vi "Listener.vi"(8 "error in (no error)":errorcluster, 11 "Hitronics in":refnum<class "Hitronics.lvclass">) -> (0 "error out":errorcluster, 2 "Buffer Dump":string, 3 "Hitronics out":refnum<class "Hitronics.lvclass">)   [LabVIEW 2018, in "Hitronics.lvlib" / "Hitronics.lvclass"]
uses:
  Hitronics.lvclass
  PPLs/Laser/Parent/Laser.lvlibp/Laser.lvclass
  C:/AME Test Engineering/LabVIEW/PPLs/Laser/Parent/Laser.lvlibp/Laser.lvclass
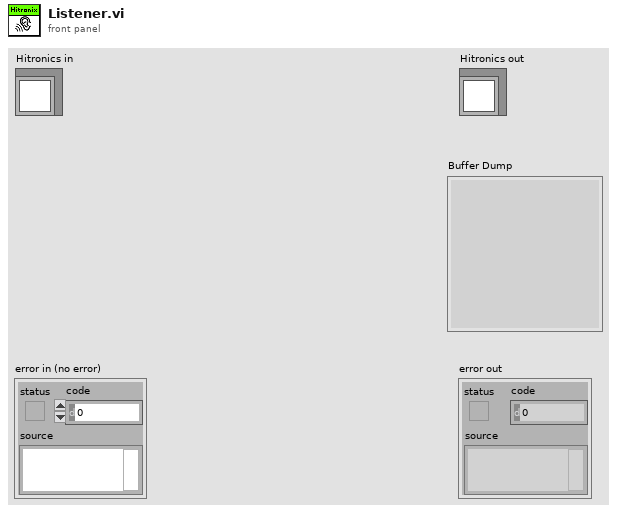
[diagram p1: front panel]
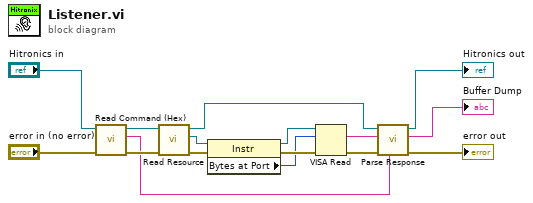
[diagram p0: block diagram]
diagram:
  n1 = call-dynamic "Read Command (Hex).vi"("error in (no error)"="error in (no error)", "Hitronics in"="Hitronics in") -> ("error out"=w13:errorcluster, "Command (Hex)"=w5:string, "Hitronics out"=w14:refnum<class "Hitronics.lvclass">)  [unwired: 7 in]
  n2 = call "Read Resource.vi"("error in (no error)"=w13, "Laser in"=w14) -> ("error out"=w12:errorcluster, "Resource"=w11:refnum<visa-resource-name>, "Laser out"=w7:refnum<class "Hitronics.lvclass">)  [unwired: 7 in]
  n3 = property class="Instr"(reference=w11, error in=w12) -> (reference out=w9:refnum<visa-resource-name>, error out=w10:errorcluster, "Bytes at Port"=w8:u32)
  n4 = VISA Read(VISA resource name=w9, byte count=w8, error in (no error)=w10) -> (read buffer=w15:string, error out=w16:errorcluster)  [unwired: 2 out]
  n5 = call "Parse Response.vi"("Command String (Hex)"=w5, "error in (no error)"=w16, "Response String (Hex)"=w15, "Hitronics in"=w7) -> ("error out"=→"error out":errorcluster, "Response"=→"Buffer Dump":string, "Hitronics out"=→"Hitronics out":refnum<class "Hitronics.lvclass">)  [unwired: 5 in]
